vi "TS_Valid_Check.vi"(11 "NewVal":T2 {"FCA" format="%01d"; "Target" min=1 max=100000; "PokaYoke" min=0 max=1}) -> (3 "Gray Out?":bool)   [LabVIEW 2020]
uses:
  Controls/TS_Parameter_V2.ctl
  <userlib>/_OpenG.lib/array/array.llb/Search 1D Array (Boolean)__ogtk.vi
  <userlib>/_OpenG.lib/array/array.llb/Index 1D Array Elements (String)__ogtk.vi
panel:
  out "length":i32[](array[numeric])
  out "output cluster":T1
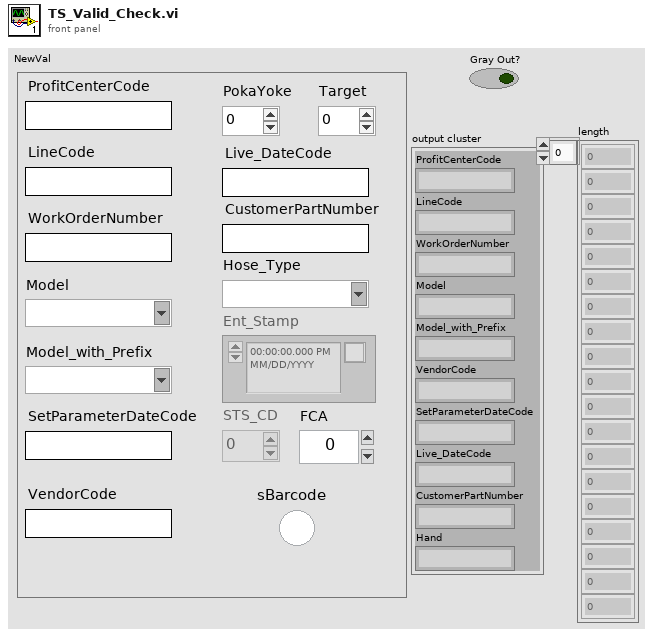
[diagram p1: front panel]
types:
  T1 = cluster{"ProfitCenterCode":string, "LineCode":string, "WorkOrderNumber":string, "Model":string, "Model_with_Prefix":string, "VendorCode":string, "SetParameterDateCode":string, "Live_DateCode":string, "CustomerPartNumber":string, "Hand":string}
  T2 = typedef "TS_Parameter_V2.ctl" = cluster{"ProfitCenterCode":string, "LineCode":string, "WorkOrderNumber":string, "Model":string, "Model_with_Prefix":string, "VendorCode":string, "SetParameterDateCode":string, "PokaYoke":i32, "Target":i32, "Live_DateCode":string, "CustomerPartNumber":string, "Hose_Type":string, "sBarcode":bool, "FCA":i32, "Ent_Stamp":timestamp, "STS_CD":dbl}
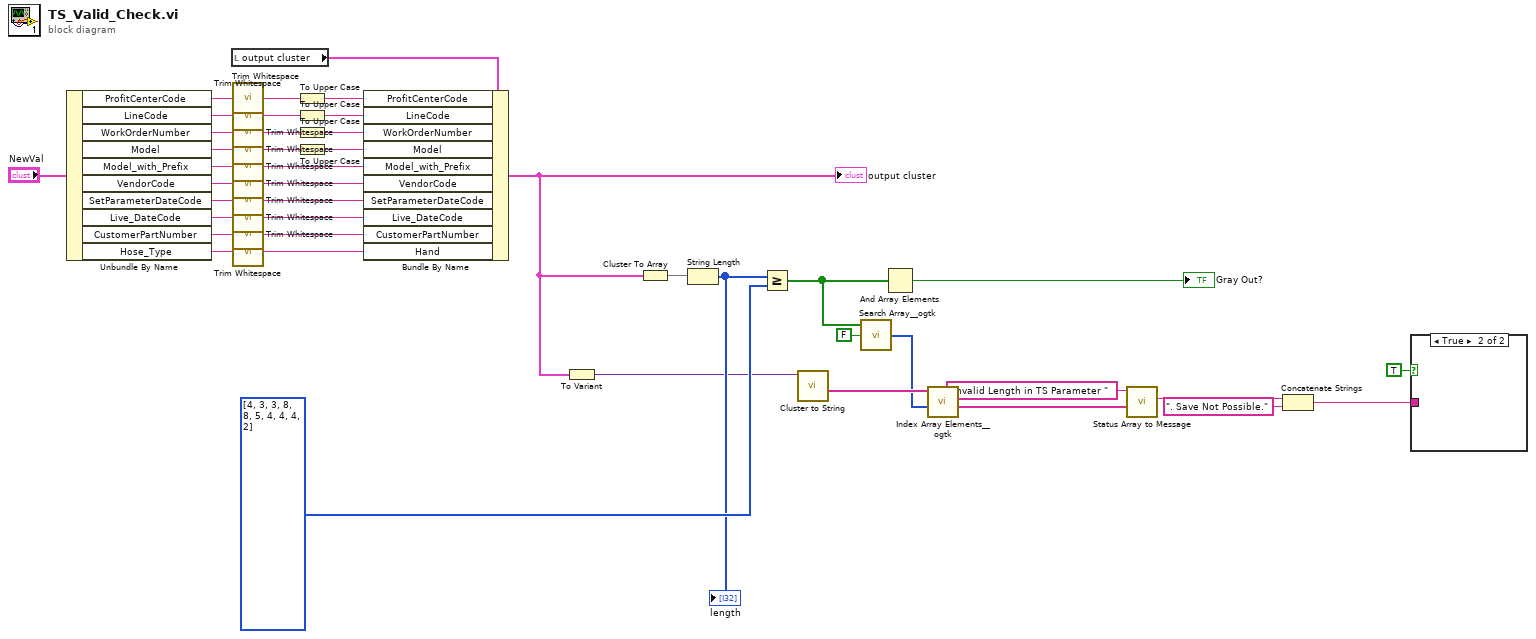
[diagram p0: block diagram]
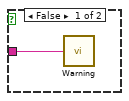
[diagram p2: hidden frame]
diagram:
  n1 = Unbundle By Name("NewVal") -> ("ProfitCenterCode"=w41:string, "LineCode"=w40:string, "WorkOrderNumber"=w39:string, "Model"=w38:string, "Model_with_Prefix"=w37:string, "VendorCode"=w36:string, "SetParameterDateCode"=w35:string, "Live_DateCode"=w34:string, "CustomerPartNumber"=w33:string, "Hose_Type"=w32:string)
  n2 = local read "output cluster"() -> (w31:T1)
  n3 = call <vilib>:"Trim Whitespace.vi"("string"=w41) -> ("trimmed string"=w15:string)  [unwired: 1 in]
  n4 = call <vilib>:"Trim Whitespace.vi"("string"=w40) -> ("trimmed string"=w13:string)  [unwired: 1 in]
  n5 = call <vilib>:"Trim Whitespace.vi"("string"=w39) -> ("trimmed string"=w11:string)  [unwired: 1 in]
  n6 = call <vilib>:"Trim Whitespace.vi"("string"=w38) -> ("trimmed string"=w10:string)  [unwired: 1 in]
  n7 = call <vilib>:"Trim Whitespace.vi"("string"=w37) -> ("trimmed string"=w9:string)  [unwired: 1 in]
  n8 = call <vilib>:"Trim Whitespace.vi"("string"=w36) -> ("trimmed string"=w8:string)  [unwired: 1 in]
  n9 = call <vilib>:"Trim Whitespace.vi"("string"=w35) -> ("trimmed string"=w7:string)  [unwired: 1 in]
  n10 = call <vilib>:"Trim Whitespace.vi"("string"=w34) -> ("trimmed string"=w6:string)  [unwired: 1 in]
  n11 = call <vilib>:"Trim Whitespace.vi"("string"=w33) -> ("trimmed string"=w5:string)  [unwired: 1 in]
  n12 = call <vilib>:"Trim Whitespace.vi"("string"=w32) -> ("trimmed string"=w4:string)  [unwired: 1 in]
  n13 = To Upper Case(1:w15) -> (0:w14:string)
  n14 = To Upper Case(1:w13) -> (0:w12:string)
  n15 = To Upper Case(1:w11) -> (0:w3:string)
  n16 = To Upper Case(1:w10) -> (0:w2:string)
  n17 = Bundle By Name(cluster=w31, "ProfitCenterCode"=w14, "LineCode"=w12, "WorkOrderNumber"=w3, "Model"=w2, "Model_with_Prefix"=w9, "VendorCode"=w8, "SetParameterDateCode"=w7, "Live_DateCode"=w6, "CustomerPartNumber"=w5, "Hand"=w4) -> (w25:T1)
  "output cluster" <- w25
  n18 = To Variant(anything=w25) -> (Variant=w16:variant)
  n19 = Cluster To Array(cluster=w25) -> (array=w30:string[])
  n20 = String Length(string=w30) -> (length=w28:i32[])
  "length" <- w28
  n21 = Greater Or Equal?(x=w28, y=i32[] [4, 3, 3, 8, 8, 5, 4, 4, 4, 2] ("length 2")) -> (x >= y?=w27:bool[])
  n22 = call <userlib>:"Cluster to String.vi"("Variant In"=w16) -> ("Format String Name"=w24:string[])  [unwired: 7 in, 3 out]
  n23 = call-poly <userlib>:"Search Array__ogtk.vi"("Array"=w27, "Element Data"=FALSE) -> ("Indices of Elements"=w23:i32[])  [unwired: 7 in]
  n24 = And Array Elements(Boolean array=w27) -> (logical AND=→"Gray Out?":bool)
  n25 = call-poly <userlib>:"Index Array Elements__ogtk.vi"("indices"=w23, "array"=w24) -> ("elements"=w22:string[])  [unwired: 9 in]
  n26 = call <userlib>:"Status Array to Message.vi"("Status Array"=w22, "Message"="Invalid Length in TS Parameter ") -> ("Message"=w20:string)  [unwired: 9 in]
  n27 = Concatenate Strings(w20, ". Save Not Possible." ("string")) -> (w19:string)
  n28 = case shown="True" TRUE {
    tunnel: w19 -> [w43 _]
    frame False {
      n29 = call <userlib>:"Warning .vi"("Warning in"=w43) -> ()  [unwired: 15 in]
    }
    frame True {
    }
  }
